vi "spec_SetOpticalExitPort.vi"(8 "error in (no error)":errorcluster, 10 "Exit Port Location":T1 items=["None"=1, "SideEntrance"=2, "FrontEntrance"=3, "SideExit"=5, "FrontExit"=4], 11 "LightField Automation in":refnum<class "LightField Automation.lvclass">) -> (0 "error out":errorcluster, 3 "LightField Automation out":refnum<class "LightField Automation.lvclass">)   [LabVIEW 2020, in "LightField Automation.lvclass"]
uses:
  LightField Automation.lvclass
  TypeDefs/OpticalPortLocation.ctl
  C:/Program Files/Princeton Instruments/LightField/PrincetonInstruments.LightFieldAddInSupportServices.dll
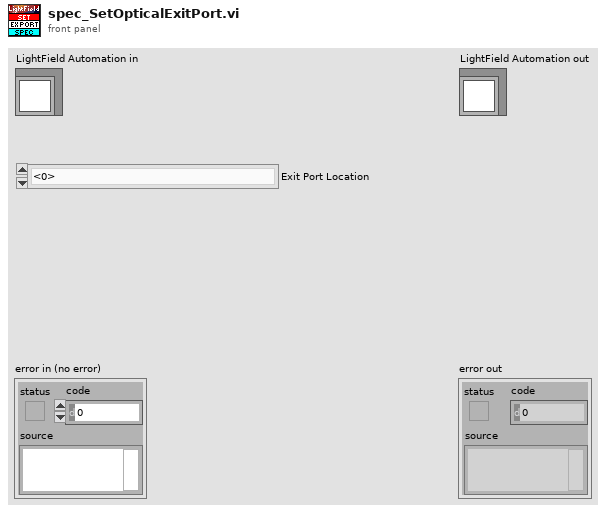
[diagram p1: front panel]
types:
  T1 = typedef "LightField Automation.lvclass/OpticalPortLocation.ctl" = i32
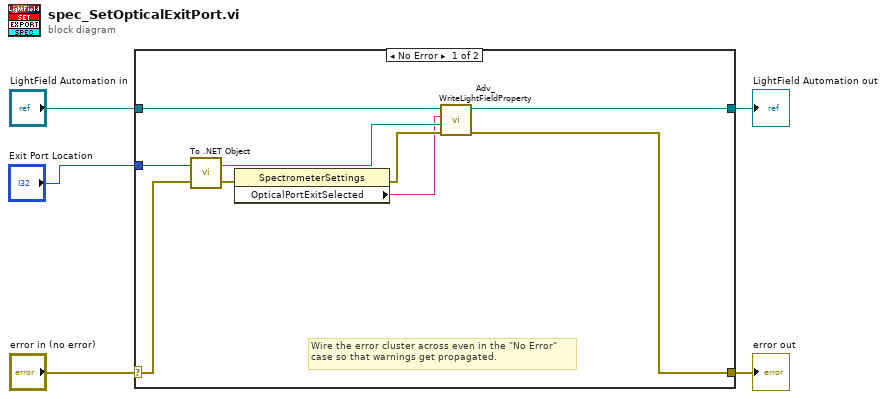
[diagram p0: block diagram]
diagram:
  n1 = case shown="No Error" "error in (no error)" {
    selector: "error in (no error)" -> [w13 w16]
    tunnel: [w8 w16] -> w4
    tunnel: [w7 w15] -> w2
    tunnel: "LightField Automation in" -> [w14 w15]
    tunnel: "Exit Port Location" -> [w6 _]
    frame No Error {
      # "Wire the error cluster across even in the \"No Error\"\ncase so that warnings get propagated."
      n2 = call <vilib>:"To .NET Object.vi"("error in (no error)"=w13, "anything"=w6) -> ("error out"=w11:errorcluster, ".NET object"=w12:refnum<k24>)
      n3 = property class="SpectrometerSettings"(error in=w11) -> (error out=w10:errorcluster, "OpticalPortExitSelected"=w9:string)  [unwired: 1 in, 1 out]
      n4 = call "Adv_WriteLightFieldProperty.vi"("error in (no error)"=w10, "value"=w12, "setting"=w9, "LightField Automation in"=w14) -> ("error out"=w8:errorcluster, "LightField Automation out"=w7:refnum<class "LightField Automation.lvclass">)  [unwired: 6 in]
    }
    frame Error {
    }
  }
  "error out" <- w4
  "LightField Automation out" <- w2
